vi "Initialize.vi"(8 "error in (no error)":errorcluster, 10 "Instrument Refnum in":refnum<visa-resource-name>, 11 "DMM in":refnum<class "DMM.lvclass">) -> (0 "error out":errorcluster, 2 "Result Text":string="PCI-4070 has been initialized", 3 "DMM out":refnum<class "DMM.lvclass">)   [LabVIEW 2012, in "DMM.lvclass"]
uses:
  DMM.lvclass
  DMM.lvclass/DMM.ctl
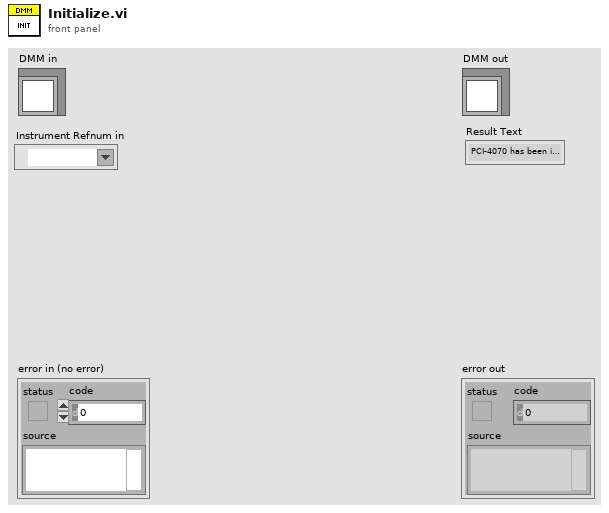
[diagram p1: front panel]
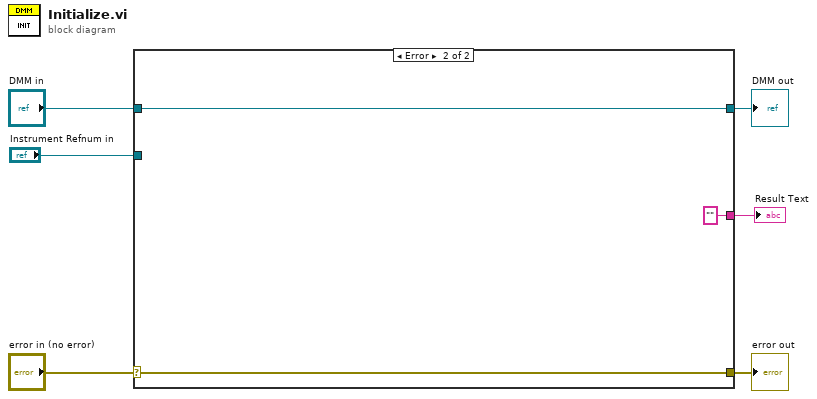
[diagram p0: block diagram]
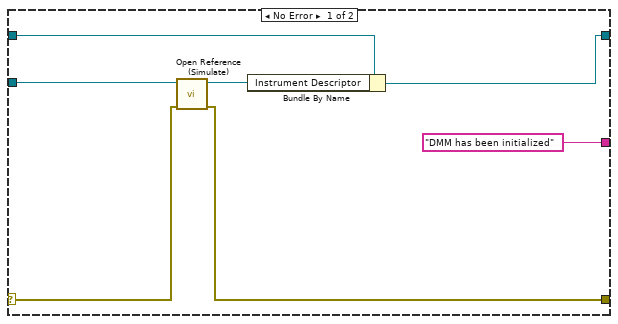
[diagram p2: hidden frame]
diagram:
  n1 = case shown="Error" "error in (no error)" {
    selector: "error in (no error)" -> [w11 w16]
    tunnel: [w10 w16] -> w5
    tunnel: [w12 w15] -> w3
    tunnel: "DMM in" -> [w13 w15]
    tunnel: "Instrument Refnum in" -> [w8 _]
    tunnel: ["DMM has been initialized" ("Result Text") "" ("Result Text")] -> w1
    frame No Error {
      n2 = call "Open Reference (Simulate).vi"("error in (no error)"=w11, "Instrument Refnum in"=w8) -> ("error out"=w10:errorcluster, "Instrument Refnum out"=w9:refnum<visa-resource-name>)  [unwired: 8 in]
      n3 = Bundle By Name(cluster=w13, "Instrument Descriptor"=w9) -> (w12:refnum<class "DMM.lvclass">)
    }
    frame Error {
    }
  }
  "error out" <- w5
  "DMM out" <- w3
  "Result Text" <- w1
